vi "Rendezvous_3_a.vi"() -> ()   [LabVIEW 2019]
uses:
  <vilib>/Platform/TimedLoop/XDataNode/timing_clust.ctl
  <vilib>/Platform/TimedLoop/XDataNode/nitl_modes.ctl
  <vilib>/Platform/TimedLoop/XDataNode/wakeup.ctl
  <vilib>/Platform/TimedLoop/scheduler/LVUserAPI/_suppVIs/Create_1kHz_TSource.vi
  <vilib>/platform/TimedLoop/XDataNode/XDataNode.xnode
  <vilib>/Platform/TimedLoop/XDataNode/XDNodeRunTimeDep.lvlib
panel:
  out "Dioda":bool
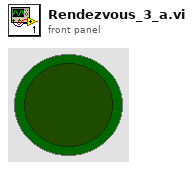
[diagram p1: front panel]
types:
  T1 = typedef "Rendezvous RefNum" = refnum<k1>
  T2 = typedef "XDNodeRunTimeDep.lvlib/timing_clust.ctl" = cluster{"Expected End [f-1]":u64, "Actual End [f-1]":u64, "Finished Late? [f-1]":bool, "Expected End [i-1]":u64, "Actual End [i-1]":u64, "Finished Late? [i-1]":bool, "Expected Start [i]":u64, "Actual Start [i]":u64, "Expected Start [f]":u64, "Actual Start [f]":u64, "Source Name":string, "Structure Name":string, "Period":i64, "Deadline":i64, "Offset":i64, "Start":i64, "Priority":i32, "Timeout":i32, "Mode":T3, "Wakeup Reason":T4, "Error":errorcluster, "Source Type":string, "Secondary Source Type":string, "Global End Time":u64, "Global Start Time":u64, "Frame Duration":u64, "Iteration Duration":u64, "Assigned CPU":i32, "I/O Scan Engine Mode":u32}
  T3 = typedef "XDNodeRunTimeDep.lvlib/nitl_modes.ctl" = enum32{"No Change", "Process missed periods, maintain original phase", "Discard missed periods, maintain original phase", "Process missed periods, ignore original phase", "Discard missed periods, ignore original phase"}
  T4 = typedef "XDNodeRunTimeDep.lvlib/wakeup.ctl" = enum32{"Normal", "Aborted", "Asynchronous wakeup", "Timing source error", "Timed loop error", "Timeout"}
  T5 = typedef "Semaphore RefNum" = refnum<k1>
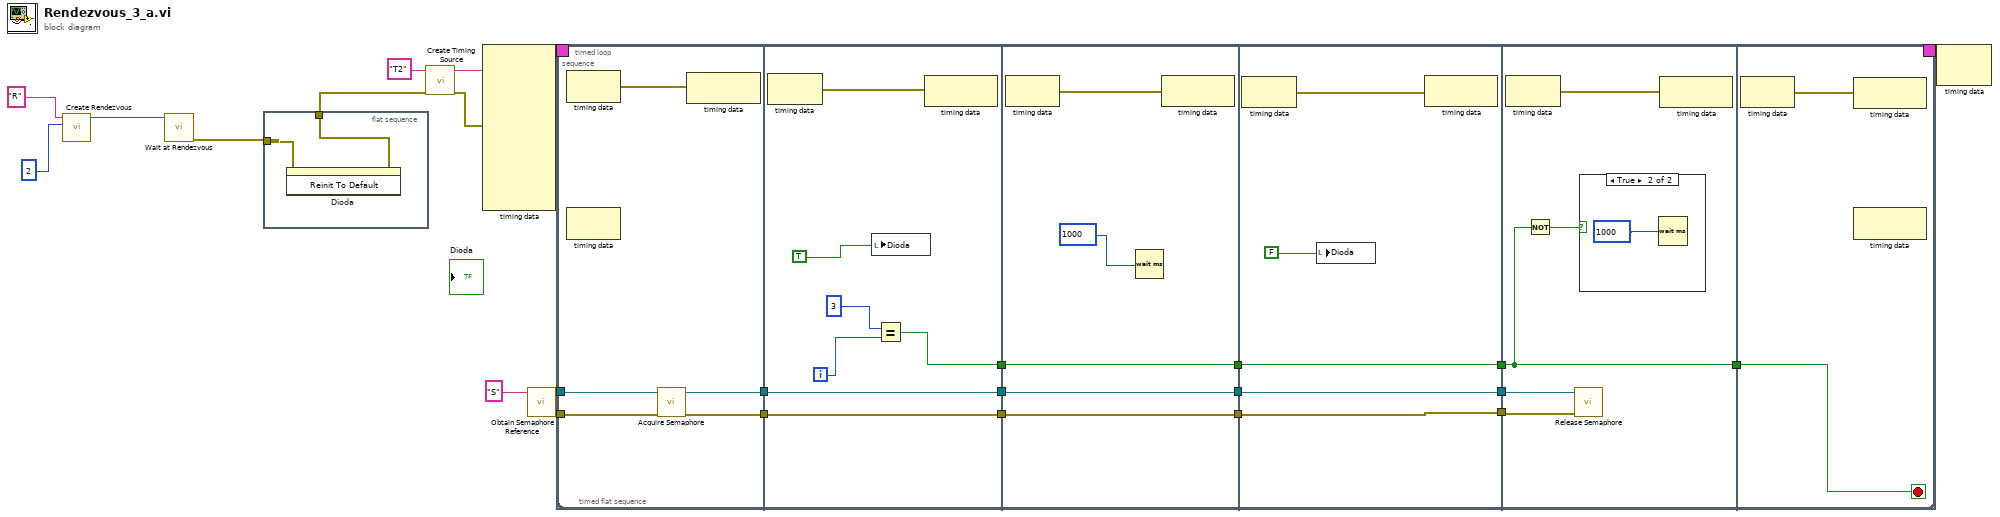
[diagram p0: block diagram]
diagram:
  n1 = call <vilib>:"Create Rendezvous.vi"("size (2)"=2, "name (unnamed)"="R") -> ("rendezvous"=w6:T1)  [unwired: 3 in, 2 out]
  n2 = call <vilib>:"Wait at Rendezvous.vi"("rendezvous"=w6) -> ("error out"=w5:errorcluster)  [unwired: 4 in, 2 out]
  n3 = flat-sequence {
    tunnel: w5 -> [w15]
    tunnel: [w14] -> w4
    frame #0 {
      n4 = invoke on="Dioda" class="Bool (strict)" method="Reinit To Default"(error in=w15) -> (error out=w14:errorcluster)  [unwired: 2 in, 2 out]
    }
  }
  n5 = call-poly <vilib>:"Create Timing Source.vi"("error in (no error)"=w4, "name (in)"="T2") -> ("error out"=w10:errorcluster, "name (out)"=w11:string)  [unwired: 8 in]
  n6 = node-c288(w11, w10) -> (w13:T2)  [unwired: 8 in]
  n7 = call <vilib>:"Obtain Semaphore Reference.vi"("name (unnamed)"="S") -> ("error out"=w1:errorcluster, "semaphore"=w2:T5)  [unwired: 4 in, 1 out]
  n8 = timed-loop {
    timing: w13 -> [_]
    timing-out: [_] -> w12
    tunnel: w2 -> [w17]
    tunnel: w1 -> [w16]
    i -> [w44]
    stop <- w86 stop-if-true
    n9 = timed-sequence {
      timing: _ -> [_]
      timing-out: _ -> [_]
      tunnel: w17 -> [w31]
      tunnel: w16 -> [w30]
      n10 = timed-flat-sequence {
        tunnel: w31 -> [w35]
        tunnel: w30 -> [w34]
        tunnel: [w33] -> w28
        tunnel: [w32] -> w26
        tunnel: [w47] -> w29
        tunnel: w28 -> [w47]
        tunnel: [w46] -> w27
        tunnel: w26 -> [w46]
        tunnel: [w42] -> w22
        tunnel: [w55] -> w25
        tunnel: w29 -> [w57]
        tunnel: w27 -> [w56]
        tunnel: [w57] -> w24
        tunnel: [w56] -> w23
        tunnel: w22 -> [w55]
        tunnel: w25 -> [w64]
        tunnel: [w64] -> w21
        tunnel: w24 -> [w67]
        tunnel: w23 -> [w66]
        tunnel: [w67] -> w19
        tunnel: [w66] -> w18
        tunnel: w21 -> [w76]
        tunnel: [w76] -> w20
        tunnel: w19 -> [w75]
        tunnel: w18 -> [w74]
        tunnel: w20 -> [w86]
        frame #0 {
          n11 = node-c288() -> (w36:errorcluster)  [unwired: 1 in]
          n12 = call <vilib>:"Acquire Semaphore.vi"("error in (no error)"=w34, "semaphore"=w35) -> ("error out"=w32:errorcluster, "semaphore out"=w33:T5)  [unwired: 3 in, 1 out]
          n13 = node-c288(w36) -> ()  [unwired: 1 out]
        }
        frame #1 {
          n14 = node-c288() -> (w48:errorcluster)  [unwired: 1 in]
          n15 = local write "Dioda"(TRUE ("LED")) -> ()
          n16 = Equal?(x=3, y=w44) -> (x = y?=w42:bool)
          n17 = node-c288(w48) -> ()  [unwired: 1 out]
        }
        frame #2 {
          n18 = node-c288() -> (w58:errorcluster)  [unwired: 1 in]
          n19 = Wait (ms)(milliseconds to wait=u32 1000) -> ()  [unwired: 1 out]
          n20 = node-c288(w58) -> ()  [unwired: 1 out]
        }
        frame #3 {
          n21 = node-c288() -> (w68:errorcluster)  [unwired: 1 in]
          n22 = local write "Dioda"(FALSE ("LED")) -> ()
          n23 = node-c288(w68) -> ()  [unwired: 1 out]
        }
        frame #4 {
          n24 = node-c288() -> (w78:errorcluster)  [unwired: 1 in]
          n25 = Not(x=w76) -> (.not. x?=w77:bool)
          n26 = call <vilib>:"Release Semaphore.vi"("error in (no error)"=w74, "semaphore"=w75) -> ()  [unwired: 4 in, 2 out]
          n27 = case shown="True" w77 {
            frame False {
            }
            frame True {
              n28 = Wait (ms)(milliseconds to wait=u32 1000) -> ()  [unwired: 1 out]
            }
          }
          n29 = node-c288(w78) -> ()  [unwired: 1 out]
        }
        frame #5 {
          n30 = node-c288() -> (w85:errorcluster)  [unwired: 1 in]
          n31 = node-c288(w85) -> ()  [unwired: 1 out]
        }
      }
    }
    n32 = node-c288() -> ()  [unwired: 1 in, 1 out]
    n33 = node-c288() -> ()  [unwired: 1 in, 1 out]
  }
  n34 = node-c288(w12) -> ()  [unwired: 1 out]
